vi "Read Path to check blacklist.vi"(11 "CDependencyInspection in":refnum<class "CDependencyInspection.lvclass">) -> (1 "Path to check blacklist":set{string}(c389), 3 "CDependencyInspection out":refnum<class "CDependencyInspection.lvclass">)   [LabVIEW 2020, in "DependencyInspection.lvlib" / "CDependencyInspection.lvclass"]
uses:
  CDependencyInspection.lvclass
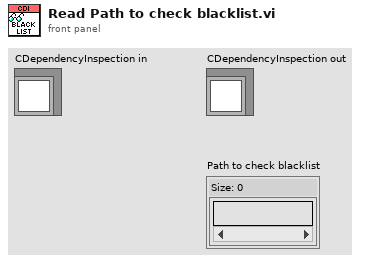
[diagram p1: front panel]
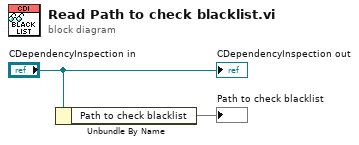
[diagram p0: block diagram]
diagram:
  n1 = Unbundle By Name("CDependencyInspection in") -> ("Path to check blacklist"=→"Path to check blacklist":set{string})
  "CDependencyInspection out" <- "CDependencyInspection in"
